vi "Gallons Adjustment.vi"(9 "Gallon Adder Input":dbl, 10 "Previous Totalizer (Gallons)":dbl, 11 "Current Totalizer (Gallons)":dbl) -> (1 "Gallon Adder Output":dbl, 3 "Normalized Gallons":dbl)   [LabVIEW 2020]
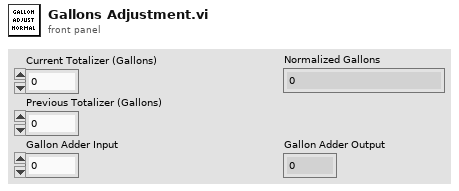
[diagram p1: front panel]
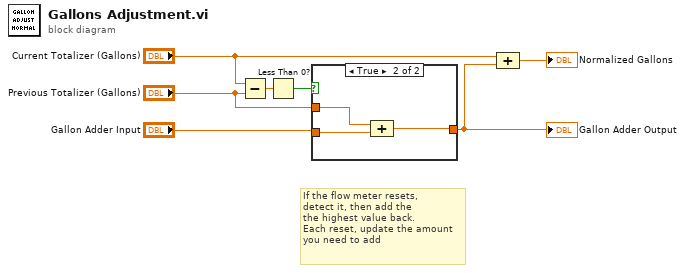
[diagram p0: block diagram]
diagram:
  # "If the flow meter resets,\ndetect it, then add the \nthe highest value back.\nEach reset, update the amount\nyou need to add"
  n1 = Subtract(x="Current Totalizer (Gallons)", y="Previous Totalizer (Gallons)") -> (x-y=w2:dbl)
  n2 = Less Than 0?(x=w2) -> (x < 0?=w4:bool)
  n3 = case shown="True" w4 {
    tunnel: "Gallon Adder Input" -> [w8 w11]
    tunnel: [w8 w10] -> w6
    tunnel: "Previous Totalizer (Gallons)" -> [_ w9]
    frame False {
    }
    frame True {
      n4 = Compound Arithmetic op=ADD(w9, w11) -> (w10:dbl)
    }
  }
  "Gallon Adder Output" <- w6
  n5 = Compound Arithmetic op=ADD("Current Totalizer (Gallons)", w6) -> (→"Normalized Gallons":dbl)
